vi "DAC Stop.vi"(11 "DevHandle":i32) -> (3 "function return":i32)   [LabVIEW 2010, in "usb2dac.lvlib"]
doc: "int WINAPI DAC_Stop(int DevHandle);"
uses:
  usb2dac.lvlib
  USB2XXX/trunk/USB2XXX/USB2XXX/vs2010/Release/USB2XXX.dll
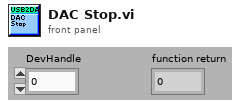
[diagram p1: front panel]
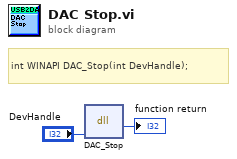
[diagram p0: block diagram]
diagram:
  # "int WINAPI DAC_Stop(int DevHandle);"
  n1 = dll-call lib="E:/Projects/USB2XXX/trunk/USB2XXX/USB2XXX/vs2010/Release/USB2XXX.*" fn="DAC_Stop"("DevHandle"="DevHandle") -> (→"function return":i32)  [unwired: 4 in, 2 out]
